vi "Create Live Random Data (Swarm).vi"(0 "Max V variatie":dbl format="%#_13g", 1 "Max H variatie":dbl format="%#_13g", 2 "TagArray In":refnum<class "Tag.lvclass">[](array[class]), 3 "AnchorArray":refnum<class "Anchor.lvclass">[](array[class]), 4 "Error margin":i32, 5 "Enable error margin":bool, 6 "DistanceLimitAnchor":dbl=150.0, 7 "SwarmInputArray":T2(array[cluster]), 8 "DistanceLimitTag":dbl=70.0 format="%#_13g", 9 "error in (no error)":errorcluster) -> (13 "error out":errorcluster, 14 "TagArray":refnum<class "Tag.lvclass">[](array[class]), 16 "AnchorArray":refnum<class "Anchor.lvclass">[](array[class]), 18 "SwarmOutputArray":T1(array[cluster]), 19 "Solution Vector":dbl[](array[numeric]) format="%.2f")   [LabVIEW 2014]
doc: "Creates random data for swarm method and solves it."
uses:
  Tag.lvclass
  Anchor/Anchor.lvclass
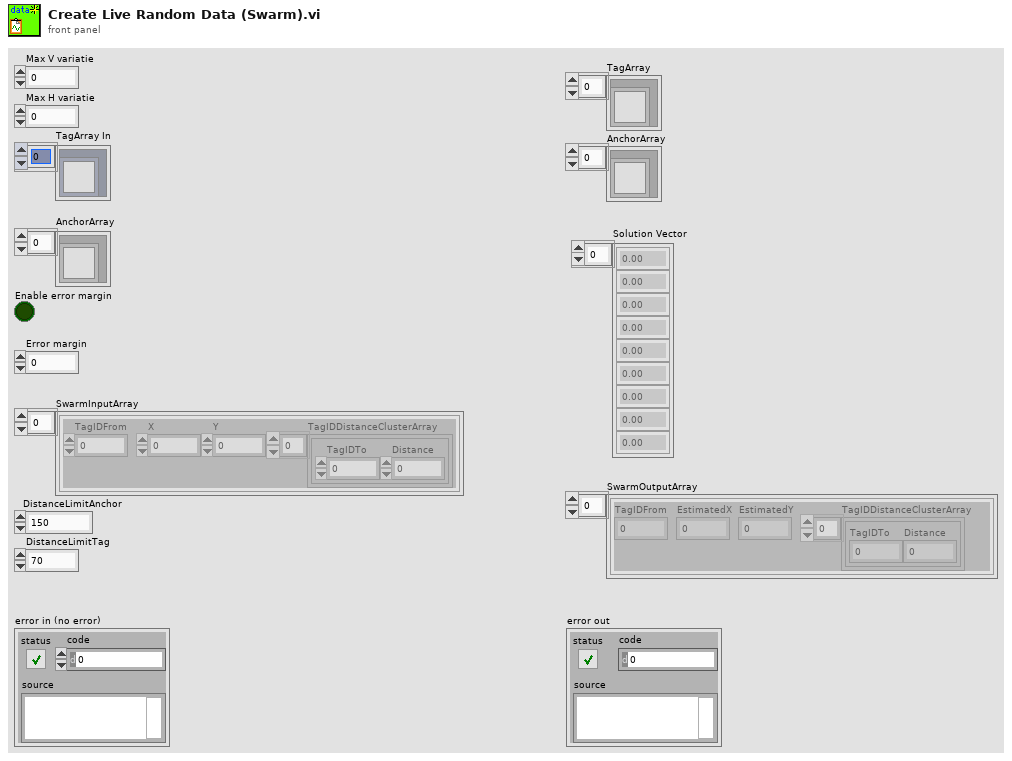
[diagram p1: front panel]
types:
  T1 = cluster{"TagIDFrom":dbl, "EstimatedX":dbl, "EstimatedY":dbl, "TagIDDistanceClusterArray":cluster{"TagIDTo":dbl, "Distance":dbl}[]}[]
  T2 = cluster{"TagIDFrom":dbl, "X":dbl, "Y":dbl, "TagIDDistanceClusterArray":cluster{"TagIDTo":dbl, "Distance":dbl}[]}[]
  T3 = cluster{"OperatingPointA":dbl, "OperatingPointB":dbl, "Tag Out":refnum<class "Tag.lvclass">}[]
  T4 = cluster{"OperatingPointA":dbl, "OperatingPointB":dbl, "Tag Out":refnum<class "Tag.lvclass">}
  T5 = cluster{"From Tag":refnum<class "Tag.lvclass">, "TagDistancesArray":cluster{"To Tag":refnum<class "Tag.lvclass">, "Tag Distance":dbl}[]}[]
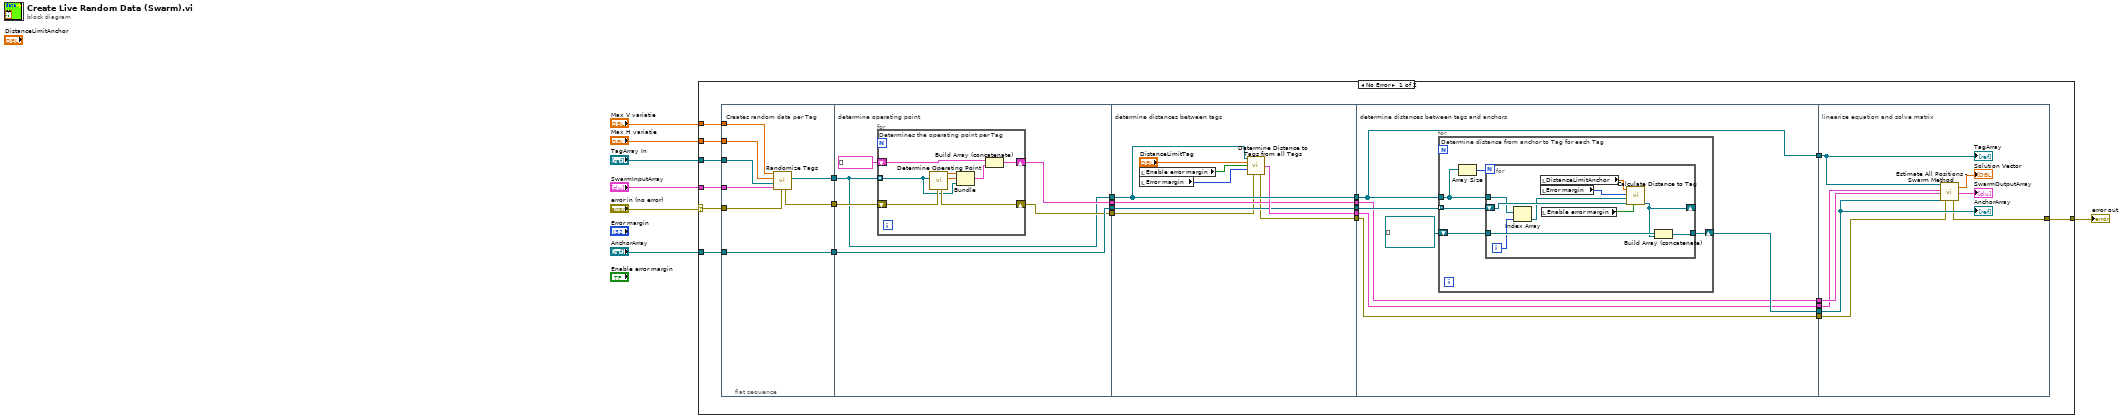
[diagram p0: block diagram]
diagram:
  n1 = case shown="No Error" "error in (no error)" {
    selector: "error in (no error)" -> [w13 w93]
    tunnel: "TagArray In" -> [w18 _]
    tunnel: "Max V variatie" -> [w17 _]
    tunnel: "Max H variatie" -> [w16 _]
    tunnel: "AnchorArray" -> [w15 _]
    tunnel: "SwarmInputArray" -> [w14 _]
    tunnel: [w8 w93] -> w1
    frame No Error {
      n2 = flat-sequence {
        tunnel: [w38] -> w31
        tunnel: [w35] -> w30
        tunnel: w18 -> [w39]
        tunnel: w17 -> [w37]
        tunnel: w16 -> [w36]
        tunnel: w15 -> [w35]
        tunnel: w14 -> [w34]
        tunnel: w13 -> [w33]
        tunnel: [w32] -> w12
        tunnel: w31 -> [w40]
        tunnel: [w40] -> w29
        tunnel: [w45] -> w28
        tunnel: w30 -> [w43]
        tunnel: [w43] -> w27
        tunnel: w12 -> [w42]
        tunnel: [w41] -> w11
        tunnel: w29 -> [w59]
        tunnel: [w59] -> w26
        tunnel: w28 -> [w57]
        tunnel: [w57] -> w25
        tunnel: w27 -> [w56]
        tunnel: [w56] -> w24
        tunnel: [w58] -> w23
        tunnel: w11 -> [w55]
        tunnel: [w54] -> w10
        tunnel: w26 -> [w69]
        tunnel: [w69] -> w22
        tunnel: w25 -> [w65]
        tunnel: [w65] -> w21
        tunnel: w24 -> [w68]
        tunnel: w23 -> [w64]
        tunnel: [w64] -> w20
        tunnel: [w67] -> w19
        tunnel: w10 -> [w63]
        tunnel: [w63] -> w9
        tunnel: w22 -> [w89]
        tunnel: w21 -> [w91]
        tunnel: w20 -> [w86]
        tunnel: w19 -> [w90]
        tunnel: w9 -> [w85]
        tunnel: [w87] -> w8
        frame #0 {
          # "Creates random data per Tag"
          n3 = call "Randomize Tags.vi"("error in (no error)"=w33, "SwarmInputArray"=w34, "TagArray In"=w39, "Max H variatie"=w36, "Max V variatie"=w37) -> ("New TagArray"=w38:refnum<class "Tag.lvclass">[], "error IO"=w32:errorcluster)  [unwired: 5 in]
        }
        frame #1 {
          # "determine operating point"
          n4 = for {
            tunnel: w40 -> [w46] mode=indexing
            shift-right: [w49] -> w45
            shift-left: T3 [] -> [w53]
            shift-right: [w47] -> w41
            shift-left: w42 -> [w48]
            # "Determines the operating point per Tag"
            n5 = call "Determine Operating Point.vi"("error in (no error)"=w48, "Tag.lvclass"=w46) -> ("OperatingPointB"=w51:dbl, "OperatingPointA"=w52:dbl, "error out"=w47:errorcluster)  [unwired: 5 in, 2 out]
            n6 = Bundle("OperatingPointA"=w52, "OperatingPointB"=w51, "Tag Out"=w46) -> (w50:T4)  [unwired: 1 in]
            n7 = Build Array (concatenate)(w53, w50) -> (w49:T3)
          }
        }
        frame #2 {
          # "determine distances between tags"
          n8 = local read "Enable error margin"() -> (w62:bool)
          n9 = local read "Error margin"() -> (w61:i32)
          n10 = call "Determine Distance to Tags from all Tags.vi"("Input TagsArray"=w59, "DistanceLimitTag"="DistanceLimitTag", "Enable Error margin?"=w62, "Error Margin"=w61, "error in (no error)"=w55) -> ("AllTagDistancesArray"=w58:T5, "error out"=w54:errorcluster)  [unwired: 9 in]
        }
        frame #3 {
          # "determine distances between tags and anchors"
          n11 = for {
            shift-right: [w74] -> w67
            shift-left: refnum<class "Anchor.lvclass">[] [] -> [w73]
            tunnel: w69 -> [w71]
            tunnel: w68 -> [w72] mode=indexing
            # "Determine distance from anchor to Tag for each Tag"
            n12 = Array Size(array=w71) -> (size(s)=w70:i32)
            n13 = for {
              N: w70 -> [_]
              tunnel: w71 -> [w78]
              shift-right: [w75] -> _
              shift-left: w72 -> [w80]
              tunnel: w73 -> [w83]
              tunnel: [w84] -> w74
              i -> [w77]
              n14 = Index Array(array=w78, index=w77) -> (element=w76:refnum<class "Tag.lvclass">)
              n15 = local read "DistanceLimitAnchor"() -> (w79:dbl)
              n16 = local read "Error margin"() -> (w81:i32)
              n17 = local read "Enable error margin"() -> (w82:bool)
              n18 = call "Calculate Distance to Tag.vi"("Enable error margin"=w82, "Anchor.lvclass In"=w80, "Tag.lvclass"=w76, "Error margin"=w81, "DistanceLimitAnchor"=w79) -> ("Anchor out"=w75:refnum<class "Anchor.lvclass">)  [unwired: 5 in, 1 out]
              n19 = Build Array (concatenate)(w83, w75) -> (w84:refnum<class "Anchor.lvclass">[])
            }
          }
        }
        frame #4 {
          # "linearize equation and solve matrix"
          n20 = call "Estimate All Positions - Swarm Method.vi"("TagArray In"=w89, "AllTagDistancesArray"=w86, "Werkpunten"=w91, "AnchorsArray"=w90, "error in (no error)"=w85) -> ("error out"=w87:errorcluster, "Solution Vector"=→"Solution Vector":dbl[], "SwarmOutputArray"=→"SwarmOutputArray":T1)  [unwired: 12 in]
          "TagArray" <- w89
          "AnchorArray" <- w90
        }
      }
    }
    frame Error {
    }
  }
  "error out" <- w1
